vi "SpectrumField3.vi"() -> ()   [LabVIEW 2024]
panel:
  in  "PauseAllDone":bool
  out "Direct Field Step:\nCurrent Value":dbl=0.1
  in  "Field Step Tab Control":enum32{"Direct Field", "Reciprocal Field"}(tab)
  in  "Direct Field Step (T)":dbl=0.1
  in  "DFS: Direct Field Step (T)":dbl=0.1
  in  "RFS: Reciprocal Field Step (1/T)":dbl=0.01
  in  "Threshold (T)":dbl=5.0
  in  "Calculate Setpoint":bool
  out "Power Supply State":string
  in  "Power Supply State":T1(ring)
  in  "Field:Rate [T/min]":dbl=0.2 min=0.0 max=0.6
  in  "Field:Final Setpoint":dbl min=-18.0 max=18.0
  out "Field: Current Value":dbl
  in  "stop":bool
  out "Field Runs":bool
  out "Field: Current Setpoint":dbl format="%.5f"
  out "Measurement Runs":bool
  in  "Steady Field":bool=TRUE
  # "Direct Field Step (DFS) will not be\nchanged below Threshold; while above: DFS=RFS*Field^2"
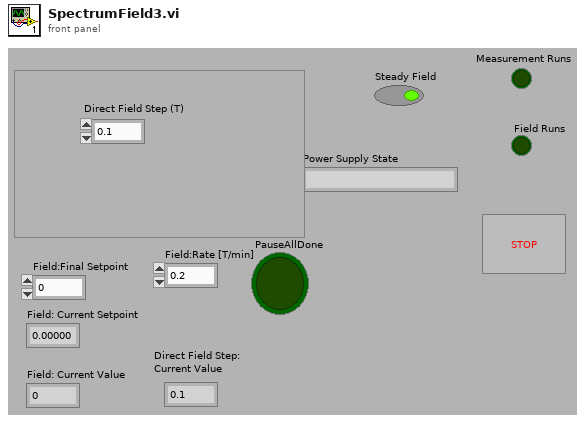
[diagram p1: front panel]
types:
  T1 = enum16{"No Response", "Ramping to programmed field ", "Holding at programmed field", "Paused", "Ramp Manual Up", "Ramp Manual Down", "Ramping to Zero", "QUENCH", "Heating Persistance Switch", "At Zero Current"}
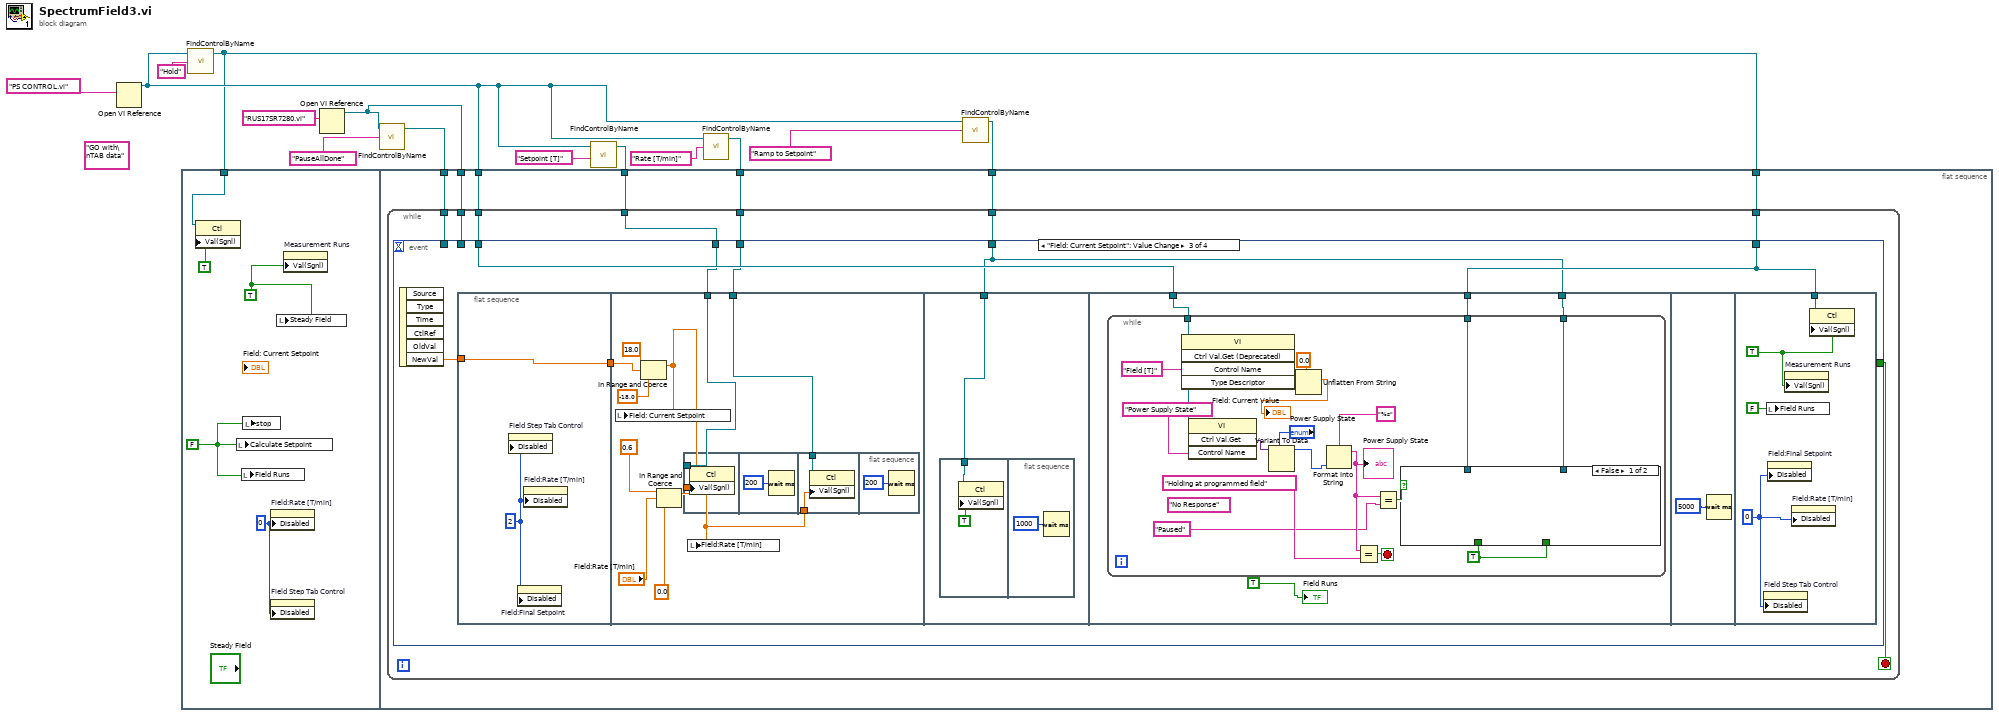
[diagram p0: block diagram]
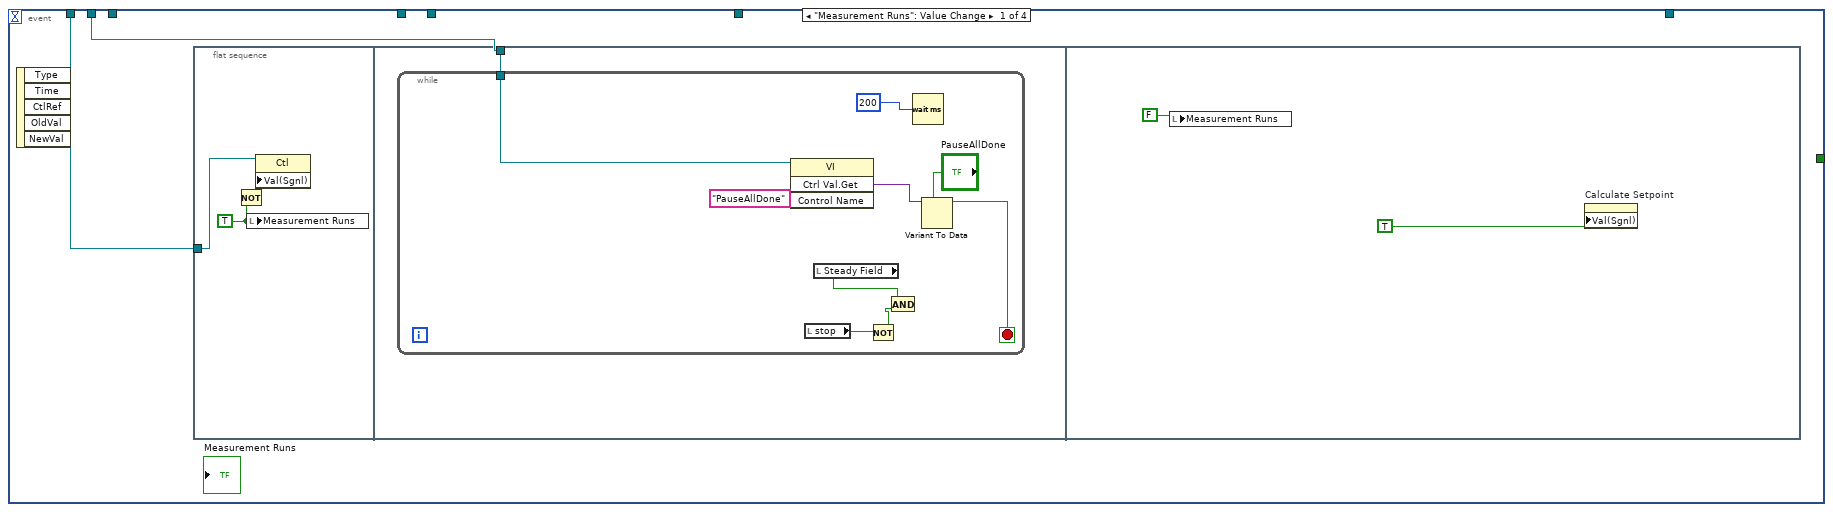
[diagram p2: hidden frame]
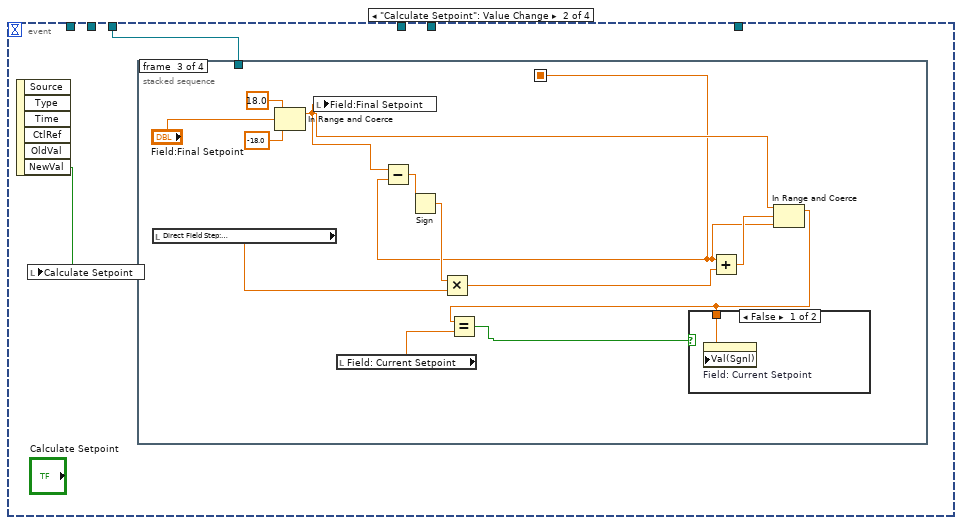
[diagram p3: hidden frame]
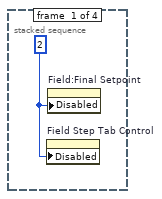
[diagram p4: hidden frame]
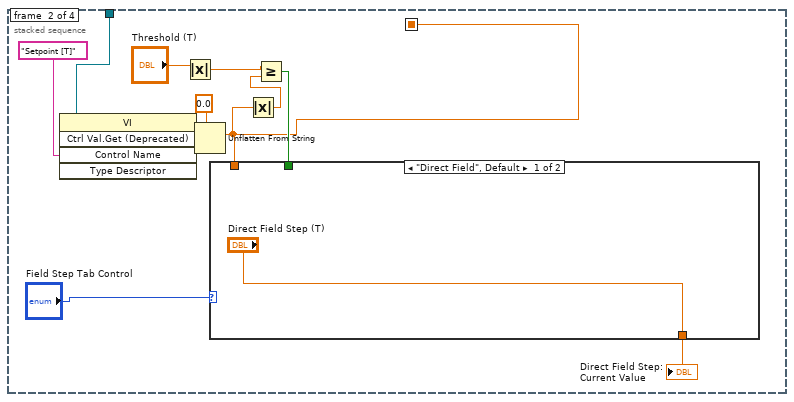
[diagram p5: hidden frame]
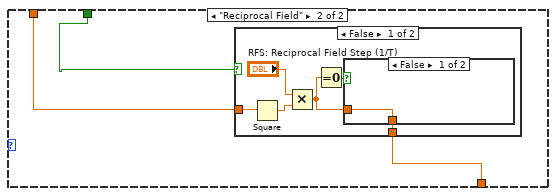
[diagram p6: hidden frame]
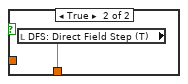
[diagram p7: hidden frame]
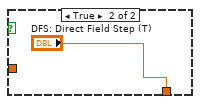
[diagram p8: hidden frame]
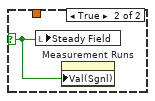
[diagram p9: hidden frame]
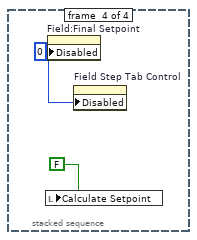
[diagram p10: hidden frame]
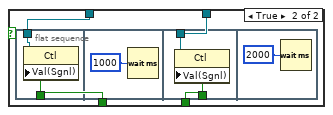
[diagram p11: hidden frame]
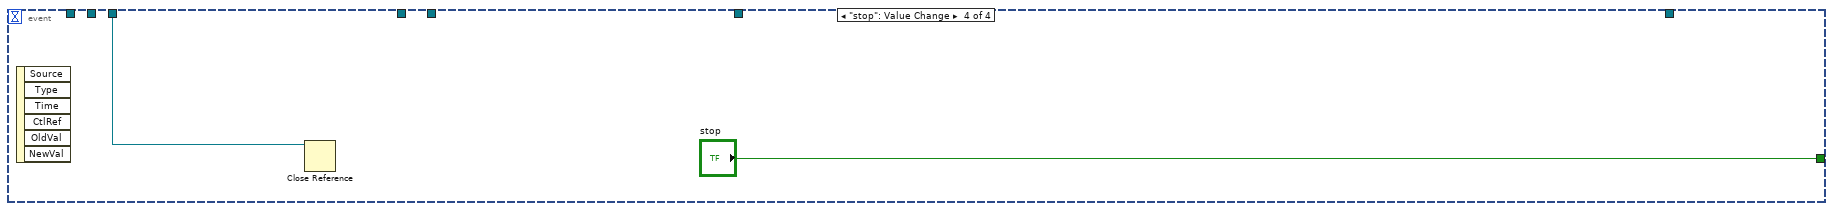
[diagram p12: hidden frame]
diagram:
  (unwired) "GO with\nTAB data" ("control name")
  n1 = Open VI Reference(vi path="PS CONTROL.vi") -> (vi reference=w6:refnum<vi>)  [unwired: 5 in, 1 out]
  n2 = flat-sequence {
    tunnel: w1 -> [w15]
    tunnel: w6 -> [w26]
    tunnel: w12 -> [w25]
    tunnel: w10 -> [w24]
    tunnel: w8 -> [w23]
    tunnel: w1 -> [w22]
    tunnel: w4 -> [w21]
    tunnel: w3 -> [w20]
    frame #0 {
      w17 = u8 0 ("Disabled")
      w19 = FALSE ("Boolean")
      w18 = TRUE ("Boolean")
      n3 = property class="Ctl"(reference=w15, "Val(Sgnl)"=TRUE ("Value (Signaling)")) -> ()  [unwired: 1 in, 2 out]
      n4 = local write "Calculate Setpoint"(w19) -> ()
      n5 = local write "Field Runs"(w19) -> ()
      n6 = local write "stop"(w19) -> ()
      n7 = property on="Field:Rate [T/min]" class="DigNum (strict)"("Disabled"=w17) -> ()  [unwired: 2 in, 2 out]
      n8 = property on="Field Step Tab Control" class="TabCtl (strict)"("Disabled"=w17) -> ()  [unwired: 2 in, 2 out]
      n9 = local write "Steady Field"(w18) -> ()
      n10 = property on="Measurement Runs" class="Bool (strict)"("Val(Sgnl)"=w18) -> ()  [unwired: 2 in, 2 out]
    }
    frame #1 {
      n11 = while {
        tunnel: w26 -> [w33]
        tunnel: w25 -> [w32]
        tunnel: w24 -> [w31]
        tunnel: w23 -> [w30]
        tunnel: w22 -> [w29]
        tunnel: w21 -> [w28]
        tunnel: w20 -> [w27]
        stop <- w34 stop-if-true
        n12 = event shown="[2] \"Field: Current Setpoint\": Value Change" {
          selector: _ -> [_ _ _ _]
          dyn-events: _ -> [_ _ _ _]
          timeout: _ -> [_ _ _ _]
          tunnel: [_ _ _ "stop"] -> w34
          tunnel: w33 -> [_ w52 w100 w162]
          tunnel: w32 -> [_ _ w99 _]
          tunnel: w31 -> [_ _ w98 _]
          tunnel: w30 -> [_ _ w96 _]
          tunnel: w29 -> [_ _ w97 _]
          tunnel: w28 -> [w36 _ _ _]
          tunnel: w27 -> [w35 _ _ _]
          event "Measurement Runs": Value Change {
            n13 = event-data() -> ()  [unwired: 1 in, 5 out]
            n14 = flat-sequence {
              tunnel: w36 -> [w38]
              tunnel: w35 -> [w40]
              frame #0 {
                w39 = TRUE ("Measurement Test")
                n15 = Not(x=w39) -> (.not. x?=w37:bool)
                n16 = local write "Measurement Runs"(w39) -> ()
                n17 = property class="Ctl"(reference=w38, "Val(Sgnl)"=w37) -> ()  [unwired: 1 in, 2 out]
              }
              frame #1 {
                n18 = while {
                  tunnel: w40 -> [w41]
                  stop <- w42 stop-if-true
                  n19 = invoke class="VI" method="Ctrl Val.Get"(reference=w41, "Control Name"="PauseAllDone") -> ("Get Control Value Variant"=w44:variant)  [unwired: 2 in, 3 out]
                  n20 = local read "stop"() -> (w48:bool)
                  n21 = local read "Steady Field"() -> (w46:bool)
                  n22 = Not(x=w48) -> (.not. x?=w47:bool)
                  n23 = And(x=w46, y=w47) -> ()  [unwired: 1 out]
                  n24 = Wait (ms)(milliseconds to wait=u32 200 ("millisecond timer value")) -> ()  [unwired: 1 out]
                  n25 = Variant To Data(type="PauseAllDone", Variant=w44) -> (data=w42:bool)  [unwired: 1 in, 1 out]
                }
              }
              frame #2 {
                n26 = local write "Measurement Runs"(FALSE ("Measurement Test")) -> ()
                n27 = property on="Calculate Setpoint" class="Bool (strict)"("Val(Sgnl)"=TRUE ("Value (Signaling)")) -> ()  [unwired: 2 in, 2 out]
              }
            }
          }
          event "Calculate Setpoint": Value Change {
            n28 = event-data() -> ("NewVal"=w53:bool)  [unwired: 1 in, 5 out]
            n29 = local write "Calculate Setpoint"(w53) -> ()
            n30 = stacked-sequence {
              seq-local: [_ w56 _ _] -> [_ _ w80 _]
              tunnel: w52 -> [_ w61 _ _]
              frame #0 {
                w54 = u8 2 ("Disabled")
                n31 = property on="Field Step Tab Control" class="TabCtl (strict)"("Disabled"=w54) -> ()  [unwired: 2 in, 2 out]
                n32 = property on="Field:Final Setpoint" class="DigNum (strict)"("Disabled"=w54) -> ()  [unwired: 2 in, 2 out]
              }
              frame #1 {
                n33 = invoke class="VI" method="Ctrl Val.Get (Deprecated)"(reference=w61, "Control Name"="Setpoint [T]") -> ("Get Control Value"=w63:string)  [unwired: 3 in, 4 out]
                n34 = Absolute Value(x="Threshold (T)") -> (abs(x)=w58:dbl)
                n35 = Unflatten From String(type=0.0, binary string=w63) -> (value=w56:dbl)  [unwired: 3 in, 2 out]
                n36 = Absolute Value(x=w56) -> (abs(x)=w59:dbl)
                n37 = Greater Or Equal?(x=w58, y=w59) -> (x >= y?=w57:bool)
                n38 = case shown="\"Direct Field\", Default" "Field Step Tab Control" {
                  tunnel: w57 -> [_ w69]
                  tunnel: w56 -> [_ w68]
                  tunnel: ["Direct Field Step (T)" w67] -> w55
                  frame "Direct Field", Default {
                  }
                  frame "Reciprocal Field" {
                    n39 = case shown="False" w69 {
                      tunnel: w68 -> [w73 _]
                      tunnel: [w70 "DFS: Direct Field Step (T)"] -> w67
                      frame False {
                        n40 = Square(x=w73) -> (x^2=w74:dbl)
                        n41 = Multiply(x="RFS: Reciprocal Field Step (1/T)", y=w74) -> (x*y=w71:dbl)
                        n42 = Equal To 0?(x=w71) -> (x = 0?=w72:bool)
                        n43 = case shown="False" w72 {
                          tunnel: w71 -> [w76 _]
                          tunnel: [w76 w77] -> w70
                          frame False {
                          }
                          frame True {
                            n44 = local read "DFS: Direct Field Step (T)"() -> (w77:dbl)
                          }
                        }
                      }
                      frame True {
                      }
                    }
                  }
                }
                "Direct Field Step:\nCurrent Value" <- w55
              }
              frame #2 {
                n45 = local read "Direct Field Step:\nCurrent Value"() -> (w79:dbl)
                n46 = In Range and Coerce(upper limit=18.0, x="Field:Final Setpoint", lower limit=-18.0) -> (coerced(x)=w81:dbl)  [unwired: 1 out]
                n47 = local write "Field:Final Setpoint"(w81) -> ()
                n48 = local read "Field: Current Setpoint"() -> (w85:dbl)
                n49 = Subtract(x=w81, y=w80) -> (x-y=w89:dbl)
                n50 = Sign(1:w89) -> (0:w88:dbl)
                n51 = Multiply(x=w88, y=w79) -> (x*y=w87:dbl)
                n52 = Add(x=w80, y=w87) -> (x+y=w86:dbl)
                n53 = In Range and Coerce(upper limit=w81, x=w86, lower limit=w80) -> (coerced(x)=w83:dbl)  [unwired: 1 out]
                n54 = Equal?(x=w83, y=w85) -> (x = y?=w84:bool)
                n55 = case shown="False" w84 {
                  selector: w84 -> [_ w93]
                  tunnel: w83 -> [w92 _]
                  frame False {
                    n56 = property on="Field: Current Setpoint" class="DigNum (strict)"("Val(Sgnl)"=w92) -> ()  [unwired: 2 in, 2 out]
                  }
                  frame True {
                    n57 = local write "Steady Field"(w93) -> ()
                    n58 = property on="Measurement Runs" class="Bool (strict)"("Val(Sgnl)"=w93) -> ()  [unwired: 2 in, 2 out]
                  }
                }
              }
              frame #3 {
                w94 = u8 0 ("Disabled")
                n59 = local write "Calculate Setpoint"(FALSE ("Calculate Setpoint")) -> ()
                n60 = property on="Field:Final Setpoint" class="DigNum (strict)"("Disabled"=w94) -> ()  [unwired: 2 in, 2 out]
                n61 = property on="Field Step Tab Control" class="TabCtl (strict)"("Disabled"=w94) -> ()  [unwired: 2 in, 2 out]
              }
            }
          }
          event "Field: Current Setpoint": Value Change {
            n62 = event-data() -> ("NewVal"=w102:dbl)  [unwired: 1 in, 5 out]
            n63 = flat-sequence {
              tunnel: w102 -> [w104]
              tunnel: [w104] -> w101
              tunnel: w101 -> [w114]
              tunnel: w99 -> [w106]
              tunnel: w98 -> [w108]
              tunnel: w96 -> [w121]
              tunnel: w100 -> [w128]
              tunnel: w97 -> [w126]
              tunnel: w96 -> [w125]
              tunnel: w97 -> [w158]
              frame #0 {
                w103 = u8 2 ("Disabled")
                n64 = property on="Field Step Tab Control" class="TabCtl (strict)"("Disabled"=w103) -> ()  [unwired: 2 in, 2 out]
                n65 = property on="Field:Final Setpoint" class="DigNum (strict)"("Disabled"=w103) -> ()  [unwired: 2 in, 2 out]
                n66 = property on="Field:Rate [T/min]" class="DigNum (strict)"("Disabled"=w103) -> ()  [unwired: 2 in, 2 out]
              }
              frame #1 {
                n67 = In Range and Coerce(upper limit=18.0, x=w114, lower limit=-18.0) -> (coerced(x)=w105:dbl)  [unwired: 1 out]
                n68 = local write "Field: Current Setpoint"(w105) -> ()
                n69 = In Range and Coerce(upper limit=0.6 ("x"), x="Field:Rate [T/min]", lower limit=0.0) -> (coerced(x)=w107:dbl)  [unwired: 1 out]
                n70 = flat-sequence {
                  tunnel: w106 -> [w116]
                  tunnel: w105 -> [w115]
                  tunnel: w108 -> [w119]
                  tunnel: w107 -> [w118]
                  frame #0 {
                    n71 = property class="Ctl"(reference=w116, "Val(Sgnl)"=w115) -> ()  [unwired: 1 in, 2 out]
                  }
                  frame #1 {
                    n72 = Wait (ms)(milliseconds to wait=u32 200 ("millisecond timer value")) -> ()  [unwired: 1 out]
                  }
                  frame #2 {
                    n73 = property class="Ctl"(reference=w119, "Val(Sgnl)"=w118) -> ()  [unwired: 1 in, 2 out]
                  }
                  frame #3 {
                    n74 = Wait (ms)(milliseconds to wait=u32 200 ("millisecond timer value")) -> ()  [unwired: 1 out]
                  }
                }
                n75 = local write "Field:Rate [T/min]"(w107) -> ()
              }
              frame #2 {
                n76 = flat-sequence {
                  tunnel: w121 -> [w122]
                  frame #0 {
                    n77 = property class="Ctl"(reference=w122, "Val(Sgnl)"=TRUE ("Value (Signaling)")) -> ()  [unwired: 1 in, 2 out]
                  }
                  frame #1 {
                    n78 = Wait (ms)(milliseconds to wait=u32 1000 ("millisecond timer value")) -> ()  [unwired: 1 out]
                  }
                }
              }
              frame #3 {
                n79 = while {
                  tunnel: w128 -> [w143]
                  tunnel: w126 -> [w131]
                  tunnel: w125 -> [w129]
                  stop <- w146 stop-if-true
                  w130 = TRUE
                  (unwired) "No Response"
                  n80 = invoke class="VI" method="Ctrl Val.Get (Deprecated)"(reference=w143, "Control Name"="Field [T]") -> ("Get Control Value"=w145:string)  [unwired: 3 in, 4 out]
                  n81 = invoke class="VI" method="Ctrl Val.Get"(reference=w143, "Control Name"="Power Supply State") -> ("Get Control Value Variant"=w139:variant)  [unwired: 2 in, 3 out]
                  n82 = Variant To Data(type="Power Supply State", Variant=w139) -> (data=w136:T1)  [unwired: 1 in, 1 out]
                  n83 = Unflatten From String(type=0.0, binary string=w145) -> (value=→"Field: Current Value":dbl)  [unwired: 3 in, 2 out]
                  n84 = Format Into String(format string="%s", w136) -> (resulting string=w134:string)  [unwired: 2 in, 1 out]
                  "Power Supply State" <- w134
                  n85 = Equal?(x=w134, y="Holding at programmed field") -> (x = y?=w146:bool)
                  n86 = Equal?(x=w134, y="Paused") -> (x = y?=w132:bool)
                  n87 = case shown="False" w132 {
                    tunnel: w131 -> [_ w150]
                    tunnel: w130 -> [_ w149]
                    tunnel: w130 -> [_ w148]
                    tunnel: w129 -> [_ w147]
                    frame False {
                    }
                    frame True {
                      n88 = flat-sequence {
                        tunnel: w150 -> [w152]
                        tunnel: w149 -> [w151]
                        tunnel: w147 -> [w155]
                        tunnel: w148 -> [w154]
                        frame #0 {
                          n89 = property class="Ctl"(reference=w152, "Val(Sgnl)"=w151) -> ()  [unwired: 1 in, 2 out]
                        }
                        frame #1 {
                          n90 = Wait (ms)(milliseconds to wait=u32 1000 ("millisecond timer value")) -> ()  [unwired: 1 out]
                        }
                        frame #2 {
                          n91 = property class="Ctl"(reference=w155, "Val(Sgnl)"=w154) -> ()  [unwired: 1 in, 2 out]
                        }
                        frame #3 {
                          n92 = Wait (ms)(milliseconds to wait=u32 2000 ("millisecond timer value")) -> ()  [unwired: 1 out]
                        }
                      }
                    }
                  }
                }
                "Field Runs" <- TRUE ("Field Test")
              }
              frame #4 {
                n93 = Wait (ms)(milliseconds to wait=u32 5000 ("millisecond timer value")) -> ()  [unwired: 1 out]
              }
              frame #5 {
                w159 = u8 0 ("Disabled")
                w160 = TRUE ("Value (Signaling)")
                n94 = property on="Field Step Tab Control" class="TabCtl (strict)"("Disabled"=w159) -> ()  [unwired: 2 in, 2 out]
                n95 = local write "Field Runs"(FALSE ("Field Test")) -> ()
                n96 = property on="Field:Final Setpoint" class="DigNum (strict)"("Disabled"=w159) -> ()  [unwired: 2 in, 2 out]
                n97 = property on="Measurement Runs" class="Bool (strict)"("Val(Sgnl)"=w160) -> ()  [unwired: 2 in, 2 out]
                n98 = property on="Field:Rate [T/min]" class="DigNum (strict)"("Disabled"=w159) -> ()  [unwired: 2 in, 2 out]
                n99 = property class="Ctl"(reference=w158, "Val(Sgnl)"=w160) -> ()  [unwired: 1 in, 2 out]
              }
            }
          }
          event "stop": Value Change {
            n100 = event-data() -> ()  [unwired: 1 in, 6 out]
            n101 = Close Reference(reference=w162) -> ()  [unwired: 1 in, 1 out]
          }
        }
      }
    }
  }
  n102 = call "FindControlByName.vi"("control name"="Hold" ("Control Name"), "vi refnum"=w6) -> ("control refnum"=w1:refnum<vi>)  [unwired: 2 in, 1 out]
  n103 = Open VI Reference(vi path="RUS17SR7280.vi") -> (vi reference=w3:refnum<vi>)  [unwired: 5 in, 1 out]
  n104 = call "FindControlByName.vi"("control name"="PauseAllDone" ("Control Name"), "vi refnum"=w3) -> ("control refnum"=w4:refnum<vi>)  [unwired: 2 in, 1 out]
  n105 = call "FindControlByName.vi"("control name"="Setpoint [T]" ("Control Name"), "vi refnum"=w6) -> ("control refnum"=w12:refnum<vi>)  [unwired: 2 in, 1 out]
  n106 = call "FindControlByName.vi"("control name"="Rate [T/min]" ("Control Name"), "vi refnum"=w6) -> ("control refnum"=w10:refnum<vi>)  [unwired: 2 in, 1 out]
  n107 = call "FindControlByName.vi"("control name"="Ramp to Setpoint" ("Control Name"), "vi refnum"=w6) -> ("control refnum"=w8:refnum<vi>)  [unwired: 2 in, 1 out]
